vi "Simulate FPGA Image Stream.vi"(10 "Image In":u8[][](array[numeric])) -> (2 "ImageVector":T1[](array[typedef]))   [LabVIEW 2015]
uses:
  <vilib>/visionFPGA/Controls/IMAQ FPGA Pixel Bus u8x1.ctl
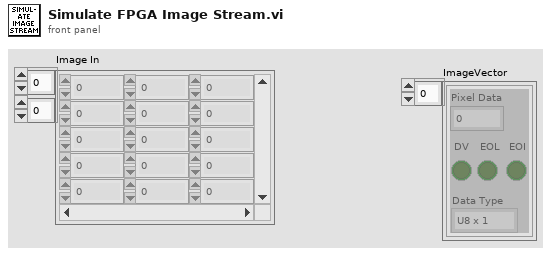
[diagram p1: front panel]
types:
  T1 = typedef "IMAQ FPGA Pixel Bus u8x1.ctl" = cluster{"Pixel Data":u8, "DV":bool, "EOL":bool, "EOI":bool, "Data Type":enum16{"U8 x 1"}}
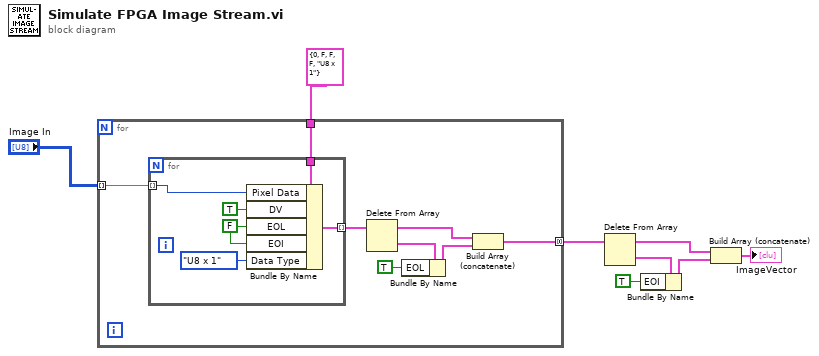
[diagram p0: block diagram]
diagram:
  n1 = for {
    tunnel: "Image In" -> [w16] mode=indexing
    tunnel: T1 {"Pixel Data"=0, "DV"=FALSE, "EOL"=FALSE, "EOI"=FALSE, "Data Type"=enum."U8 x 1"} ("Hue Plane Out") -> [w15]
    tunnel: [w9] -> w2 mode=concatenating
    n2 = for {
      tunnel: w16 -> [w21] mode=indexing
      tunnel: w15 -> [w22]
      tunnel: [w19] -> w14 mode=indexing
      w17 = FALSE ("EOL")
      n3 = Bundle By Name(cluster=w22, "Pixel Data"=w21, "DV"=TRUE, "EOL"=w17, "EOI"=w17, "Data Type"=enum16{"U8 x 1"}."U8 x 1") -> (w19:T1)
    }
    n4 = Delete From Array(array=w14) -> (deleted portion=w13:T1, array with subset deleted=w11:T1[])  [unwired: 2 in]
    n5 = Bundle By Name(cluster=w13, "EOL"=TRUE) -> (w10:T1)
    n6 = Build Array (concatenate)(w11, w10) -> (w9:T1[])
  }
  n7 = Delete From Array(array=w2) -> (deleted portion=w3:T1, array with subset deleted=w5:T1[])  [unwired: 2 in]
  n8 = Bundle By Name(cluster=w3, "EOI"=TRUE ("EOL")) -> (w6:T1)
  n9 = Build Array (concatenate)(w5, w6) -> (→"ImageVector":T1[])
